vi "TCP ENGINE Async Data JSON Conversion.vi"(8 "error in":errorcluster, 11 "JSON String":string) -> (0 "error out":errorcluster, 1 "Data":variant, 2 "SubCmd":string, 3 "Command":string)   [LabVIEW 2018, in "TCP Engine.lvlib"]
doc: "All Rights Reserved © 2017 SyncSols"
uses:
  TCP Engine.lvlib
  Controls/JSON Async Configure3.ctl
  Controls/JSON ARINC Start.ctl
  Controls/JSON Async Message.ctl
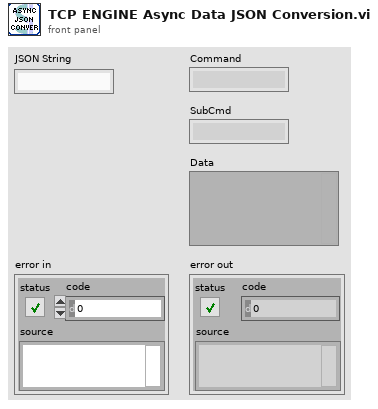
[diagram p1: front panel]
types:
  T1 = typedef "TCP Engine.lvlib/JSON Async Message.ctl" = cluster{"Command":string, "SubCmd":string, "Data":cluster{"Port":string, "MsgLength":i32, "Data":i32[]}}
  T2 = typedef "TCP Engine.lvlib/JSON ARINC Start.ctl" = cluster{"Command":string, "SubCmd":string, "Data":string}
  T3 = typedef "TCP Engine.lvlib/JSON Async Configure3.ctl" = cluster{"Command":string, "SubCmd":string, "Data":cluster{"Port":string, "Baud":i32, "Databits":i32, "Parity":i32, "Stopbits":i32, "Flowcontrol":i32}[]}
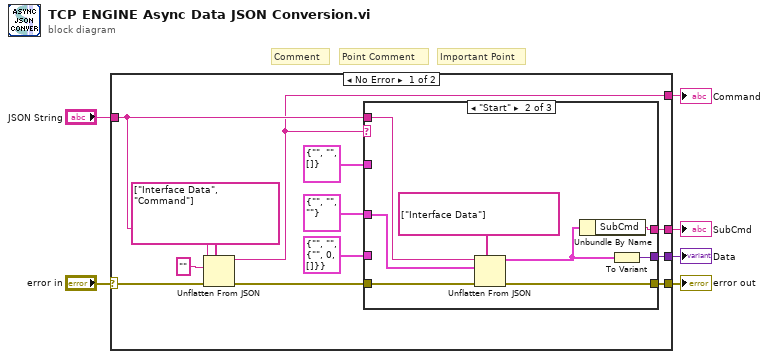
[diagram p0: block diagram]
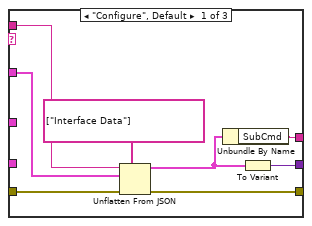
[diagram p2: hidden frame]
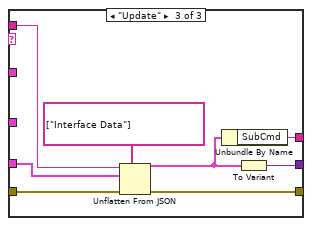
[diagram p3: hidden frame]
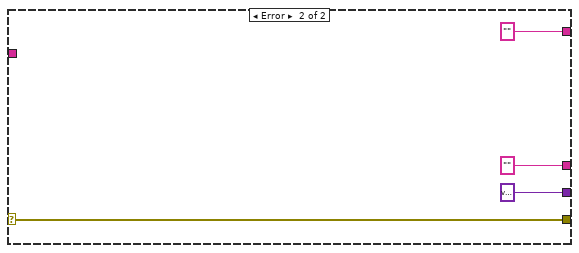
[diagram p4: hidden frame]
diagram:
  # "Important Point"
  # "Point Comment"
  # "Comment"
  n1 = case shown="No Error" "error in" {
    selector: "error in" -> [w18 w46]
    tunnel: [w13 w46] -> w6
    tunnel: "JSON String" -> [w15 _]
    tunnel: [w12 "" ("SubCmd")] -> w3
    tunnel: [w11 ""] -> w2
    tunnel: [w10 variant ("Variant")] -> w1
    frame No Error {
      n2 = Unflatten From JSON(path=string[] ["Interface Data", "Command"], JSON string=w15, type and defaults="", error in (no error)=w18) -> (value=w11:string, error out=w14:errorcluster)  [unwired: 3 in]
      n3 = case shown="\"Start\"" w11 {
        tunnel: T3 {"Command"="", "SubCmd"="", "Data"=[]} -> [w25 _ _]
        tunnel: w15 -> [w24 w33 w41]
        tunnel: T2 {"Command"="", "SubCmd"="", "Data"=""} -> [_ w32 _]
        tunnel: w14 -> [w23 w31 w40]
        tunnel: [w22 w30 w39] -> w13
        tunnel: [w21 w29 w38] -> w10
        tunnel: [w19 w27 w36] -> w12
        tunnel: T1 {"Command"="", "SubCmd"="", "Data"={"Port"="", "MsgLength"=0, "Data"=[]}} ("value") -> [_ _ w35]
        frame "Configure", Default {
          n4 = Unflatten From JSON(path=string[] ["Interface Data"], JSON string=w24, type and defaults=w25, error in (no error)=w23) -> (value=w20:T3, error out=w22:errorcluster)  [unwired: 3 in]
          n5 = Unbundle By Name(w20) -> ("SubCmd"=w19:string)
          n6 = To Variant(anything=w20) -> (Variant=w21:variant)
        }
        frame "Start" {
          n7 = Unflatten From JSON(path=string[] ["Interface Data"], JSON string=w33, type and defaults=w32, error in (no error)=w31) -> (value=w28:T2, error out=w30:errorcluster)  [unwired: 3 in]
          n8 = Unbundle By Name(w28) -> ("SubCmd"=w27:string)
          n9 = To Variant(anything=w28) -> (Variant=w29:variant)
        }
        frame "Update" {
          n10 = Unflatten From JSON(path=string[] ["Interface Data"], JSON string=w41, type and defaults=w35, error in (no error)=w40) -> (value=w37:T1, error out=w39:errorcluster)  [unwired: 3 in]
          n11 = Unbundle By Name(w37) -> ("SubCmd"=w36:string)
          n12 = To Variant(anything=w37) -> (Variant=w38:variant)
        }
      }
    }
    frame Error {
    }
  }
  "error out" <- w6
  "SubCmd" <- w3
  "Command" <- w2
  "Data" <- w1
